vi "test 呼吸同不.vi"() -> ()   [LabVIEW 2011]
uses:
  <vilib>/Waveform/DWDTOps.llb/DWDT Boolean Array to Digital.vi
panel:
  out "数字波形图":digitalwaveform(graph)
  out "port1（5元素）":bool[](array[boolean])
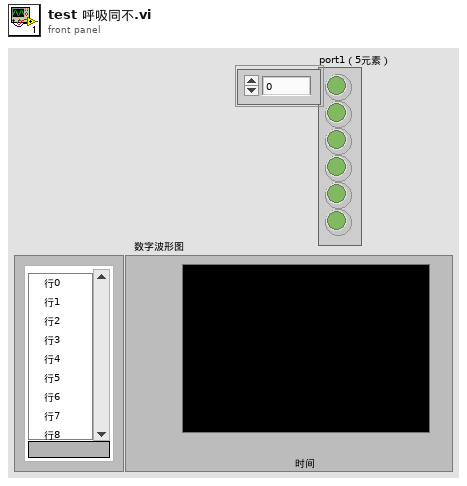
[diagram p1: front panel]
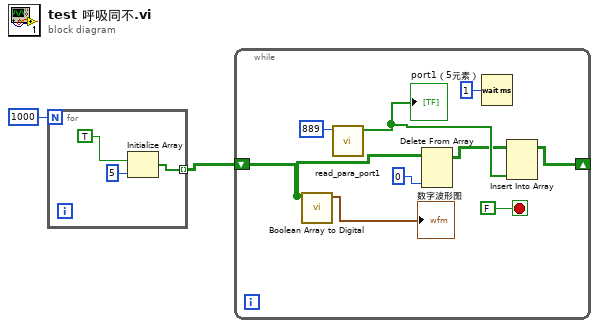
[diagram p0: block diagram]
diagram:
  n1 = for {
    N: 1000 -> [_]
    tunnel: [w3] -> w2 mode=indexing
    n2 = Initialize Array(TRUE, 5 ("维数大小")) -> (w3:bool[])
  }
  n3 = while {
    shift-right: [w8] -> _
    shift-left: w2 -> [w10]
    stop <- FALSE stop-if-true
    n4 = call-poly <vilib>:"Boolean Array to Digital.vi"("boolean array"=w10) -> ("digital waveform"=→"数字波形图":digitalwaveform)  [unwired: 9 in, 1 out]
    n5 = call "read_para_port1.vi"("address"=i16 889) -> ("port1（5元素）"=w9:bool[])  [unwired: 9 in, 1 out]
    "port1（5元素）" <- w9
    n6 = Delete From Array(array=w10, index (col)=0 ("禁用的索引 (列)")) -> (array with subset deleted=w6:bool[][])  [unwired: 2 in, 1 out]
    n7 = Wait (ms)(milliseconds to wait=u32 1 ("等待时间（毫秒）")) -> ()  [unwired: 1 out]
    n8 = Insert Into Array(array=w6, new element=w9) -> (w8:bool[][])  [unwired: 2 in]
  }
